vi "Trans In.vi"(1 "消息数据":variant, 3 "消息":string) -> (0 "输出簇":T1)   [LabVIEW 2023]
uses:
  Ctl/QMH Fundamentals - Message Cluster.ctl
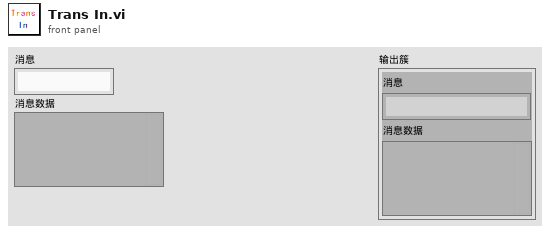
[diagram p1: front panel]
types:
  T1 = typedef "QMH Fundamentals - Message Cluster.ctl" = cluster{"消息":string, "消息数据":variant}
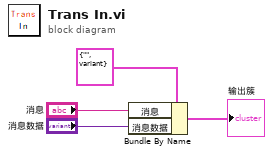
[diagram p0: block diagram]
diagram:
  n1 = Bundle By Name(cluster=T1 {"消息"="", "消息数据"=variant} ("Message Cluster"), "消息"="消息", "消息数据"="消息数据") -> (→"输出簇":T1)
